vi "Com_SECS Equipment _Stream_S1F14.vi"(8 "error in":errorcluster, 11 "S1F14 Setting":T1) -> (0 "error out":errorcluster, 3 "SECS Packet":T2)   [LabVIEW 2016]
uses:
  Data Def/Com_SECS Equipment _SECS Packet.ctl
  Data Def/Com_SECS Equipment _Message Type.ctl
  Data Def/Com_SECS Equipment _Protocol Type.ctl
  Data Def/Com_SECS Equipment _Stream Type.ctl
  Data Def/Com_SECS Equipment _Build Message Setting.ctl
  Data Message/Com_SECS Equipment _Data Message_List.vi
  Data Message/Com_SECS Equipment _Data Message_ASCII.vi
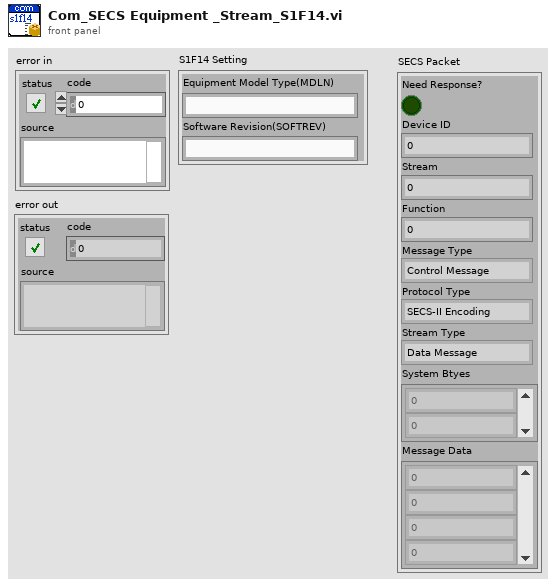
[diagram p1: front panel]
types:
  T1 = cluster{"Equipment Model Type(MDLN)":string, "Software Revision(SOFTREV)":string}
  T2 = typedef "Com_SECS Equipment _SECS Packet.ctl" = cluster{"Need Response?":bool, "Device ID":u16, "Stream":u8, "Function":u8, "Message Type":T3, "Protocol Type":T4, "Stream Type":T5, "System Btyes":u8[], "Message Data":u8[]}
  T3 = typedef "Com_SECS Equipment _Message Type.ctl" = enum16{"Control Message", "Data Message"}
  T4 = typedef "Com_SECS Equipment _Protocol Type.ctl" = enum16{"SECS-II Encoding", "Reserved"}
  T5 = typedef "Com_SECS Equipment _Stream Type.ctl" = enum16{"Data Message", "Select.req", "Select.rsp", "Deselect.req", "Deselect.rsp", "Linktest.req", "Linktest.rsp", "Reject.req", "Separate.req", "Reserve"}
  T6 = typedef "Com_SECS Equipment _Build Message Setting.ctl" = cluster{"Stream":u8, "Function":u8, "Need Response?":bool}
  T7 = typedef "Com_SECS Equipment _Message Data.ctl" = cluster{"Index":i32, "Data Item Format":T8, "Format Code":T9, "Parent Index":i32, "Child Index":i32[], "Data":variant}
  T8 = typedef "Com_SECS Equipment _Data Item Format.ctl" = enum16{"Data Type", "Value"}
  T9 = typedef "Com_SECS Equipment _Format Code.ctl" = enum16{"L", "A", "B", "Boolean", "J", "I1", "I2", "I4", "I8", "U1", "U2", "U4", "U8", "F4", "F8", "Char"}
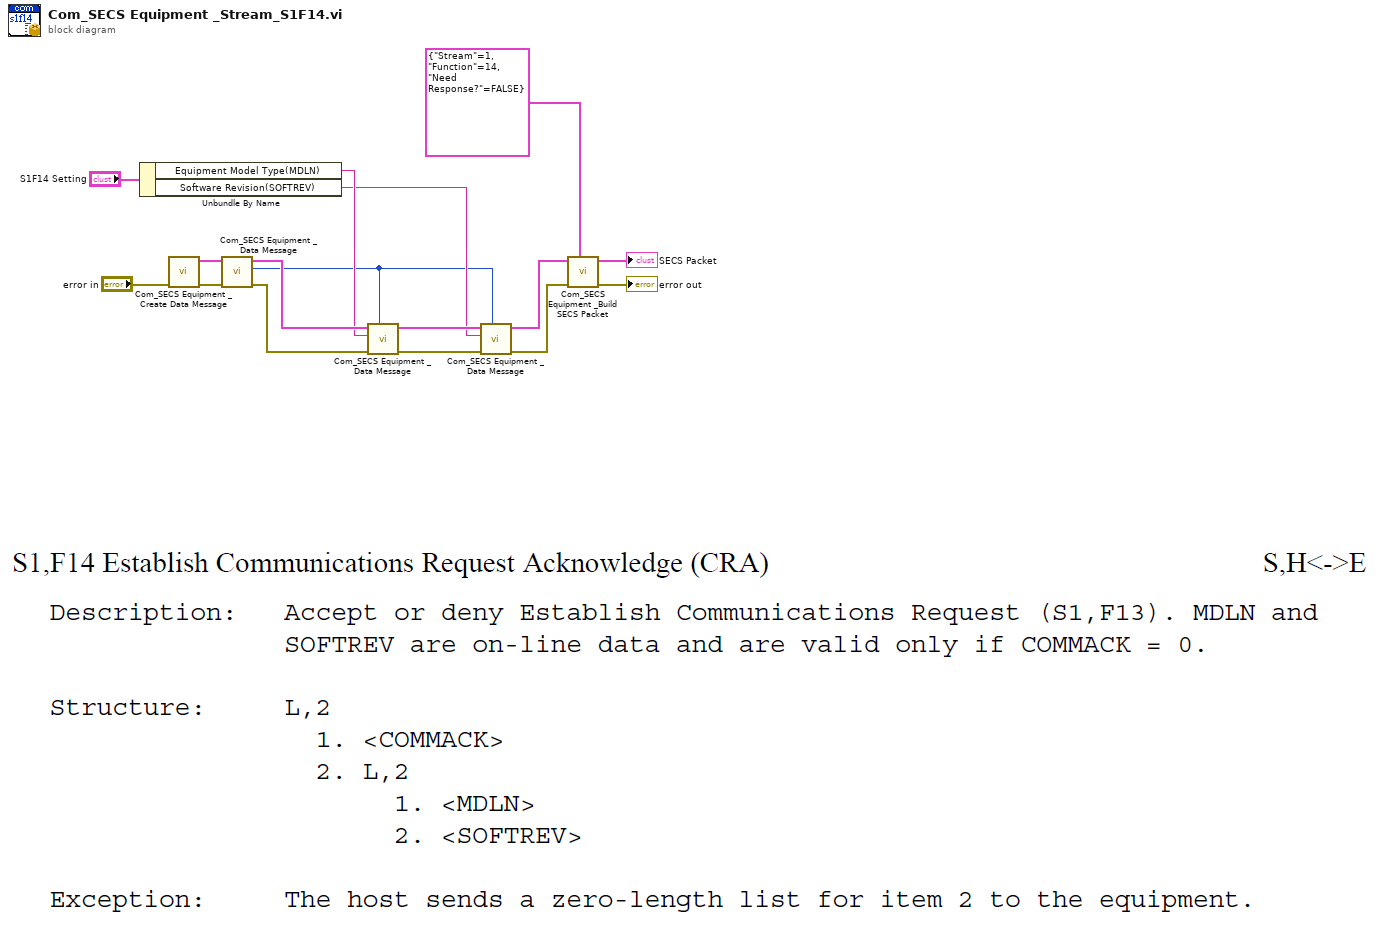
[diagram p0: block diagram]
diagram:
  n1 = Unbundle By Name("S1F14 Setting") -> ("Equipment Model Type(MDLN)"=w7:string, "Software Revision(SOFTREV)"=w4:string)
  n2 = call "Com_SECS Equipment _Create Data Message.vi"("error in"="error in") -> ("error out"=w12:errorcluster, "Message Data"=w11:T7[])  [unwired: 9 in]
  n3 = call-poly "Com_SECS Equipment _Data Message.vi"("error in"=w12, "Message Data In"=w11) -> ("error out"=w10:errorcluster, "Index"=w3:i32, "Message Data Out"=w9:T7[])  [unwired: 7 in]
  n4 = call-poly "Com_SECS Equipment _Data Message.vi"("Parent Index"=w3, "error in"=w10, "Data"=w7, "Message Data In"=w9) -> ("error out"=w6:errorcluster, "Message Data Out"=w5:T7[])  [unwired: 6 in]
  n5 = call-poly "Com_SECS Equipment _Data Message.vi"("Parent Index"=w3, "error in"=w6, "Data"=w4, "Message Data In"=w5) -> ("error out"=w2:errorcluster, "Message Data Out"=w1:T7[])  [unwired: 6 in]
  n6 = call "Com_SECS Equipment _Build SECS Packet.vi"("Build Message Setting"=T6 {"Stream"=1, "Function"=14, "Need Response?"=FALSE}, "error in"=w2, "Message Data"=w1) -> ("error out"=→"error out":errorcluster, "SECS Packet"=→"SECS Packet":T2)  [unwired: 7 in]
